vi "Move DC_1_Power.vi"(2 "DC Motor":cluster{"DC Motor":T2, "Address":i16}={"DC Motor"=enum."DC Motor", "Address"=-1}, 3 "NXT":T1={"Hardware"="NXT", "Flattened String"=""}, 4 "Power (100)":i8=100) -> (0 "NXT":T1={"Hardware"="NXT", "Flattened String"=""})   [LabVIEW 2010, in "4134Outputs.lvlib"]
uses:
  4134Outputs.lvlib
  <vilib>/NXT/Subs/MotorXNode.DC Motor Type.ctl
  <vilib>/NXT/Subs/LVHSConnector.ctl
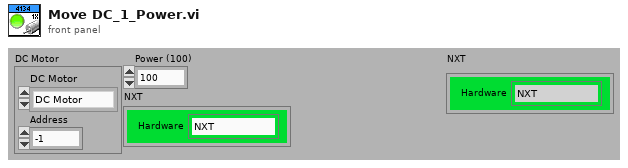
[diagram p1: front panel]
types:
  T1 = typedef "LVHSConnector.ctl" = cluster{"Hardware":string, "Flattened String":string}
  T2 = typedef "MotorXNode.DC Motor Type.ctl" = enum16{"DC Motor"}
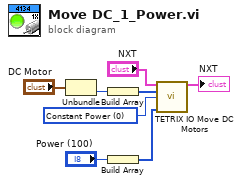
[diagram p0: block diagram]
diagram:
  w3 = u8 0 items=["Constant Power", "Constant Speed"] ("Control Mode (Constant Power)")
  n1 = Unbundle("DC Motor") -> ("Address"=w7:i16)  [unwired: 1 out]
  n2 = Build Array(w7) -> (w6:i16[])
  n3 = Build Array("Power (100)") -> (w4:i8[])
  n4 = call <vilib>:"TETRIX IO Move DC Motors.vi"("NXT"="NXT", "DC Motors"=w6, "Control Mode (Constant Power)"=w3, "Power / Speed"=w4) -> ("NXT"=→"NXT":T1)  [unwired: 11 in]
